vi "Sensirion SHT25 - VISA read.vi"(8 "Error In":errorcluster, 11 "VISA in":refnum<visa-resource-name>) -> (0 "Error Out":errorcluster, 1 "humidity":dbl, 2 "temperature":dbl, 3 "VISA out":refnum<visa-resource-name>)   [LabVIEW 2012]
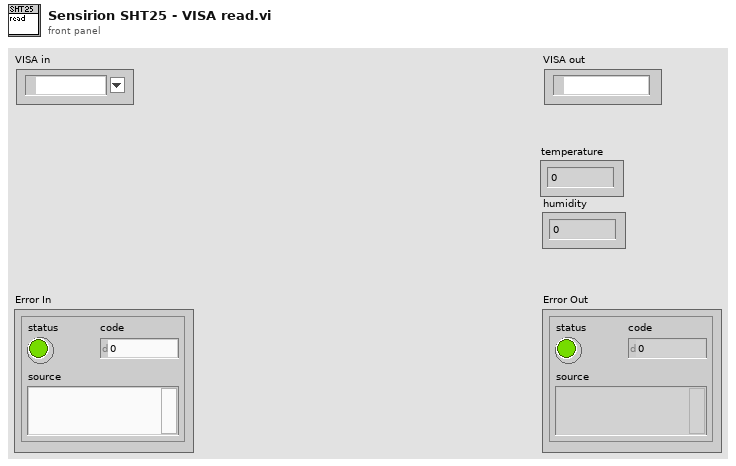
[diagram p1: front panel]
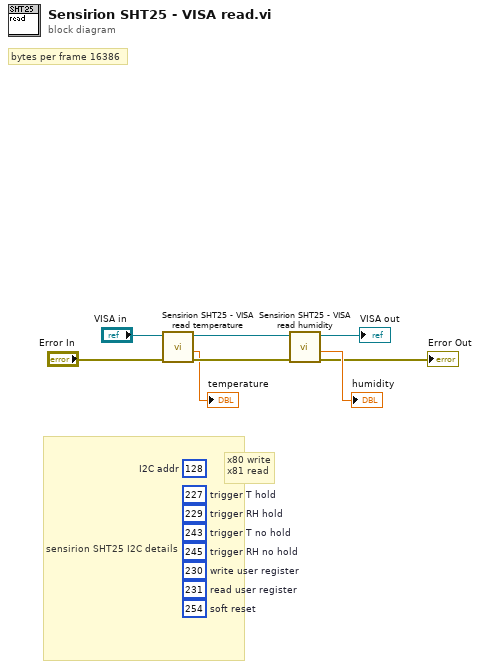
[diagram p0: block diagram]
diagram:
  (unwired) u8 254  # soft reset
  (unwired) u8 231  # read user register
  (unwired) u8 230  # write user register
  (unwired) u8 245  # trigger RH no hold
  (unwired) u8 243  # trigger T no hold
  (unwired) u8 229  # trigger RH hold
  (unwired) u8 128  # I2C addr
  (unwired) u8 227  # trigger T hold
  # "x80 write\nx81 read"
  # "bytes per frame 16386"
  # "sensirion SHT25 I2C details"
  n1 = call "Sensirion SHT25 - VISA read temperature.vi"("Error In"="Error In", "VISA in"="VISA in") -> ("Error Out"=w5:errorcluster, "temperature"=→"temperature":dbl, "VISA out"=w6:refnum<visa-resource-name>)  [unwired: 7 in]
  n2 = call "Sensirion SHT25 - VISA read humidity.vi"("Error In"=w5, "VISA in"=w6) -> ("Error Out"=→"Error Out":errorcluster, "humidity"=→"humidity":dbl, "VISA out"=→"VISA out":refnum<visa-resource-name>)  [unwired: 7 in]
